vi "Cleanup.vi"(8 "error in (no error)":errorcluster, 11 "Stop Bug Remover in":refnum<class "Stop Air Dry.lvclass">) -> (0 "error out":errorcluster, 3 "Stop Bug Remover out":refnum<class "Stop Air Dry.lvclass">)   [LabVIEW 2019, in "Stop Air Dry.lvclass"]
uses:
  <vilib>/gpm_packages/@cs/Car-wash/Source/Process Steps/Stop Air Dry/Stop Air Dry.lvclass
  <vilib>/gpm_packages/@cs/Car-wash/Source/iProcess Step Model/iProcess Step Model/iProcess Step Model.lvclass
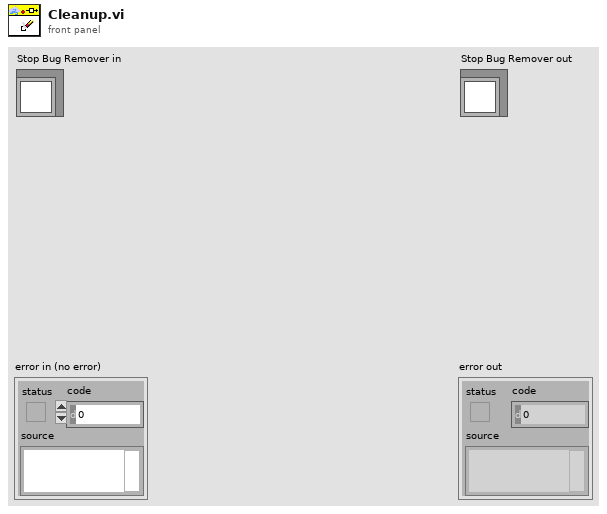
[diagram p1: front panel]
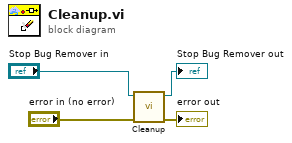
[diagram p0: block diagram]
diagram:
  n1 = call-parent "Cleanup.vi"("error in (no error)"="error in (no error)", "iProcess Step Model in"="Stop Bug Remover in") -> ("error out"=→"error out":errorcluster, "iProcess Step Model out"=→"Stop Bug Remover out":refnum<class "Stop Air Dry.lvclass">)  [unwired: 8 in]
